vi "Ventus - Update Power.vi"(4 "error in (no error)":errorcluster, 5 "Power (%)":dbl, 6 "VISA resource name":refnum<visa-resource-name>) -> (0 "error out":errorcluster, 2 "VISA resource name out":refnum<visa-resource-name>)   [LabVIEW 2020]
panel:
  out "return count":u32
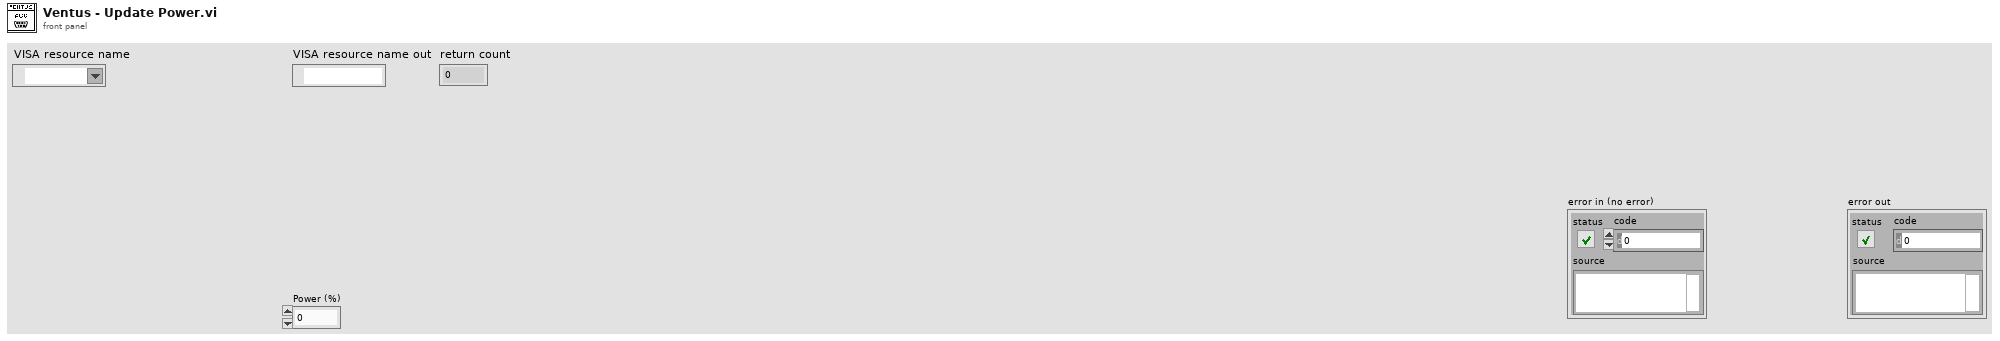
[diagram p1: front panel]
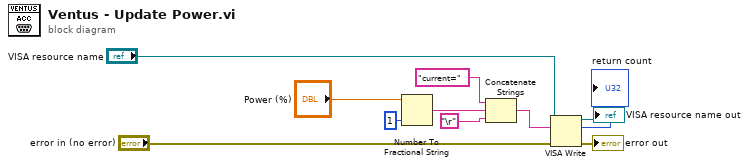
[diagram p0: block diagram]
diagram:
  n1 = Number To Fractional String(number="Power (%)", precision (6)=i16 1) -> (F-format string=w8:string)  [unwired: 2 in]
  n2 = Concatenate Strings("current=", w8, "\r") -> (w10:string)
  n3 = VISA Write(VISA resource name="VISA resource name", write buffer=w10, error in (no error)="error in (no error)") -> (VISA resource name out=→"VISA resource name out":refnum<visa-resource-name>, return count=→"return count":u32, error out=→"error out":errorcluster)
